vi "Response 7265.vi"(8 "error in (no error)":errorcluster, 11 "7265 GPIB":string="7") -> (0 "error out":errorcluster={"status"=TRUE, "code"=6, "source"="GPIB Read in Command and Response 7265.vi"}, 1 "Response Description":string, 2 "Response Code Only":dbl format="%#_7p", 3 "Response":string)   [LabVIEW 2014]
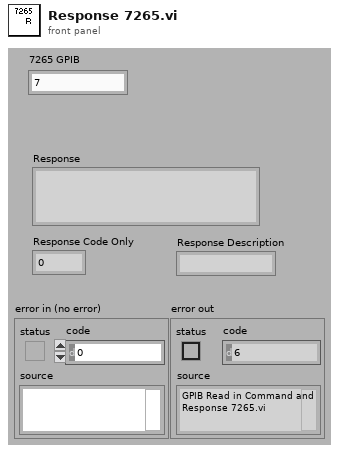
[diagram p1: front panel]
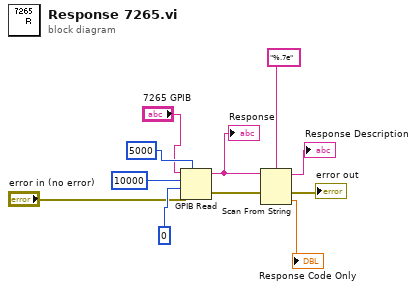
[diagram p0: block diagram]
diagram:
  n1 = GPIB Read(0:"7265 GPIB", 1:10000 ("timeout ms (488.2 global)"), 2:i16 0 ("mode (0)"), 3:"error in (no error)", 4:5000 ("timeout ms (488.2 global)")) -> (5:w8:string, 7:w7:errorcluster)  [unwired: 1 out]
  "Response" <- w8
  n2 = Scan From String(format string="%.7e", input string=w8, error in=w7) -> (remaining string=→"Response Description":string, error out=→"error out":errorcluster, output 1=→"Response Code Only":dbl)  [unwired: 2 in, 1 out]
